vi "BasicErrorLogger.vi"(2 "error in":errorcluster, 3 "indicator":refnum<vi>) -> (0 "error out":errorcluster, 1 "recent":string[](array[string]))   [LabVIEW 2012]
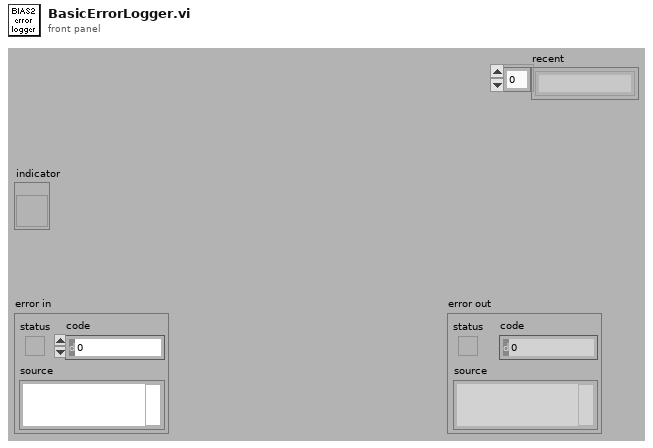
[diagram p1: front panel]
types:
  T1 = cluster{"status":bool, "code":i32, "description":string, "time":timestamp}
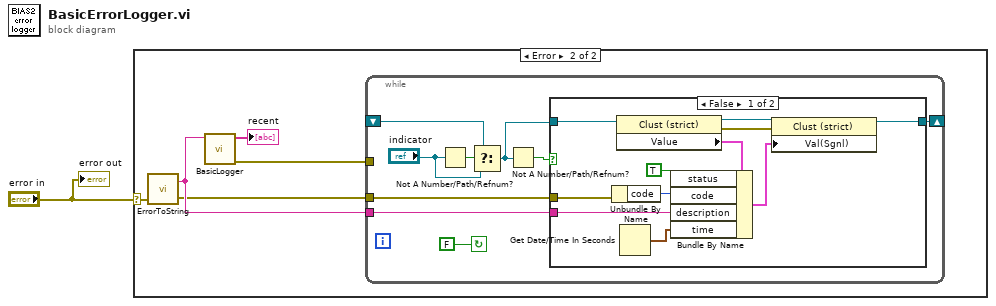
[diagram p0: block diagram]
diagram:
  n1 = case shown="Error" "error in" {
    selector: "error in" -> [_ w4]
    frame No Error {
    }
    frame Error {
      n2 = call <userlib>:"ErrorToString.vi"("error in (no error)"=w4) -> ("error out"=w2:errorcluster, "error string"=w5:string)  [unwired: 1 in]
      n3 = call <userlib>:"BasicLogger.vi"("text"=w5) -> ("error out"=w3:errorcluster, "recent"=→"recent":string[])  [unwired: 6 in]
      n4 = while {
        shift-right: [w11] -> _
        shift-left: _ -> [w14]
        tunnel: w2 -> [w8]
        tunnel: w5 -> [w9]
        tunnel: w3 -> [_]
        stop <- FALSE continue-if-true
        n5 = Not A Number/Path/Refnum?(number/path/refnum="indicator") -> (NaN/Path/Refnum?=w15:bool)
        n6 = Select(t=w14, s=w15, f="indicator") -> (s? t:f=w12:refnum<vi>)
        n7 = Not A Number/Path/Refnum?(number/path/refnum=w12) -> (NaN/Path/Refnum?=w7:bool)
        n8 = case shown="False" w7 {
          tunnel: w12 -> [w26 w27]
          tunnel: [w25 w27] -> w11
          tunnel: w9 -> [w24 _]
          tunnel: w8 -> [w23 _]
          frame False {
            n9 = Unbundle By Name(w23) -> ("code"=w16:i32)
            n10 = property class="Clust (strict)"(reference=w26) -> (reference out=w20:refnum<vi>, error out=w19:errorcluster, "Value"=w21:T1)  [unwired: 1 in]
            n11 = Get Date/Time In Seconds() -> (seconds since 1Jan1904=w17:timestamp)
            n12 = Bundle By Name(cluster=w21, "status"=TRUE, "code"=w16, "description"=w24, "time"=w17) -> (w22:T1)
            n13 = property class="Clust (strict)"(reference=w20, error in=w19, "Val(Sgnl)"=w22) -> (reference out=w25:refnum<vi>)  [unwired: 1 out]
          }
          frame True {
          }
        }
      }
    }
  }
  "error out" <- "error in"
